vi "Tosca-Editor.vi"(0 "Tosca":refnum<class "Parameters.lvclass">, 2 "Parent VI":refnum<vi>, 5 "FSM In":refnum<class "FSM.Graph.lvclass">, 9 "Cal Folder":path) -> (4 "Tosca out":refnum<class "Parameters.lvclass">, 6 "FSM out":refnum<class "FSM.Graph.lvclass">, 10 "canceled":bool)   [LabVIEW 2020]
uses:
  FSM Graph VIs/LV Source/FSM Editor/FSM Editor.xctl
  FSM Graph VIs/LV Source/Classes/FSM.Graph/FSM.Graph.lvclass
  Controls/Timeout XCtrl/Timeout XCtrl.xctl
  Classes/Timeout/Timeout.lvclass
  Controls/TTL XCtrl/TTL XCtrl.xctl
  Classes/Parameters/Parameters.lvclass
  Controls/Input Event XCtrl/Input Event XCtrl.xctl
  epl-vi-lib/Utility VIs/Controls/KTable/KTable.xctl
  epl-vi-lib/Utility VIs/Controls/KListboxEx/KListboxEx.xctl
  Controls/Termination XCtrl/Termination XCtrl.xctl
  Classes/Termination/Termination.lvclass
  epl-vi-lib/Signal Synthesis VIs/4th Generation/Controls/SignalManager/SignalManager.xctl
  epl-vi-lib/Signal Synthesis VIs/4th Generation/Classes/SignalManager/SignalManager.lvclass
  Classes/Parameters/Parameters.lvclass/Parameters.ctl
  Typedefs/Tosca-Schedule Mode.ctl
  Classes/State/State.lvclass/State.ctl
  FSM Graph VIs/LV Source/Classes/FSM.Node/Badge.ctl
  epl-vi-lib/Signal Synthesis VIs/4th Generation/Classes/SignalManager/SignalManager.lvclass/SignalManager.ctl
  Classes/Timeout/Timeout.lvclass/Timeout.ctl
  Classes/Termination/Termination.lvclass/Termination.ctl
  Classes/Parameters/Read Flowchart.vi
  Classes/Parameters/Write DAQ.vi
  Classes/Parameters/Write Schedule Mode.vi
  Classes/Parameters/Read Input Events.vi
  Classes/Parameters/Read Flags.vi
  Classes/State/Read Name.vi
  Classes/Parameters/Write First state.vi
  Classes/Parameters/Write Target state.vi
  epl-vi-lib/Signal Synthesis VIs/4th Generation/Classes/SignalManager/Read Fs (Hz).vi
  Classes/Parameters/Read Pretrial.vi
  Classes/Parameters/Read DAQ.vi
  Classes/Parameters/Read Schedule Mode.vi
  Classes/State/Read Timeouts.vi
  Classes/Timeout/Read Link to.vi
  Classes/Timeout/Read Type.vi
  epl-vi-lib/Signal Synthesis VIs/4th Generation/Classes/SignalManager/Read Error.vi
  Classes/State/Read script.vi
  Classes/State/Read TTL-only.vi
  Classes/State/Read SigMan.vi
  Classes/State/Read Grating.vi
  Classes/Parameters/Read First state.vi
  Classes/Parameters/Read Target state.vi
  Classes/Timeout/Read TTL.vi
  Classes/State/Read Term.vi
  Classes/Termination/Read TTL.vi
  Classes/Termination/Read Source.vi
  Classes/Termination/Read Type.vi
  Sub VIs/Tosca-Globals.vi
  Classes/State/State.lvclass
  TTL VIs/Control Classes/Base Class/TTLController.lvclass
  FSM Graph VIs/LV Source/Classes/FSM.Node/FSM.Node.lvclass
panel:
  in  "Template":u16(ring) items=["Create from template...", "Basic"]
  in  "FSM.Graph":refnum<class "FSM.Graph.lvclass">(xcontrol)
  in  "Cancel":bool
  in  "Apply":bool
  in  "Tabs":T1(tab)
  in  "icon":u16(ring)
  in  "Mode":u16(ring) caption="Configure as" items=["Sequence", "CS+/CS-", "Adaptive track"]
  in  "DAQ":T2
  in  "Input Event":T6(xcontrol)
  in  "Flags":u16(xcontrol)
  in  "EventList":i32(xcontrol) caption="Input event..."
  in  "State.Script":bool caption="Re-execute script"
  in  "Time/Term":enum32{"Timeout", "Term"}(tab)
  in  "Timeout":refnum<class "Timeout.lvclass">(xcontrol)
  in  "Term":refnum<class "Termination.lvclass">(xcontrol) caption="Lick"
  in  "State.Target":bool caption="Target state"
  in  "State.Start here":bool caption="Start here"
  in  "State.Name":string caption="Name"
  in  "TTL":refnum<class "TTLController.lvclass">[](xcontrol)
  in  "SigMan":refnum<class "SignalManager.lvclass">(xcontrol)
  in  "Sig Tab":enum32{"Error", "Plot"}(tab)
  out "Error":string
  out "Graph":dbl[][](graph)
  in  "Grating":T7
  in  "Test Button":bool
  # "delay between starting locomotion tracking, \nSynapse, etc. and before starting first trial"
  # "Events evaluated in this order.\nDrag to rearrange"
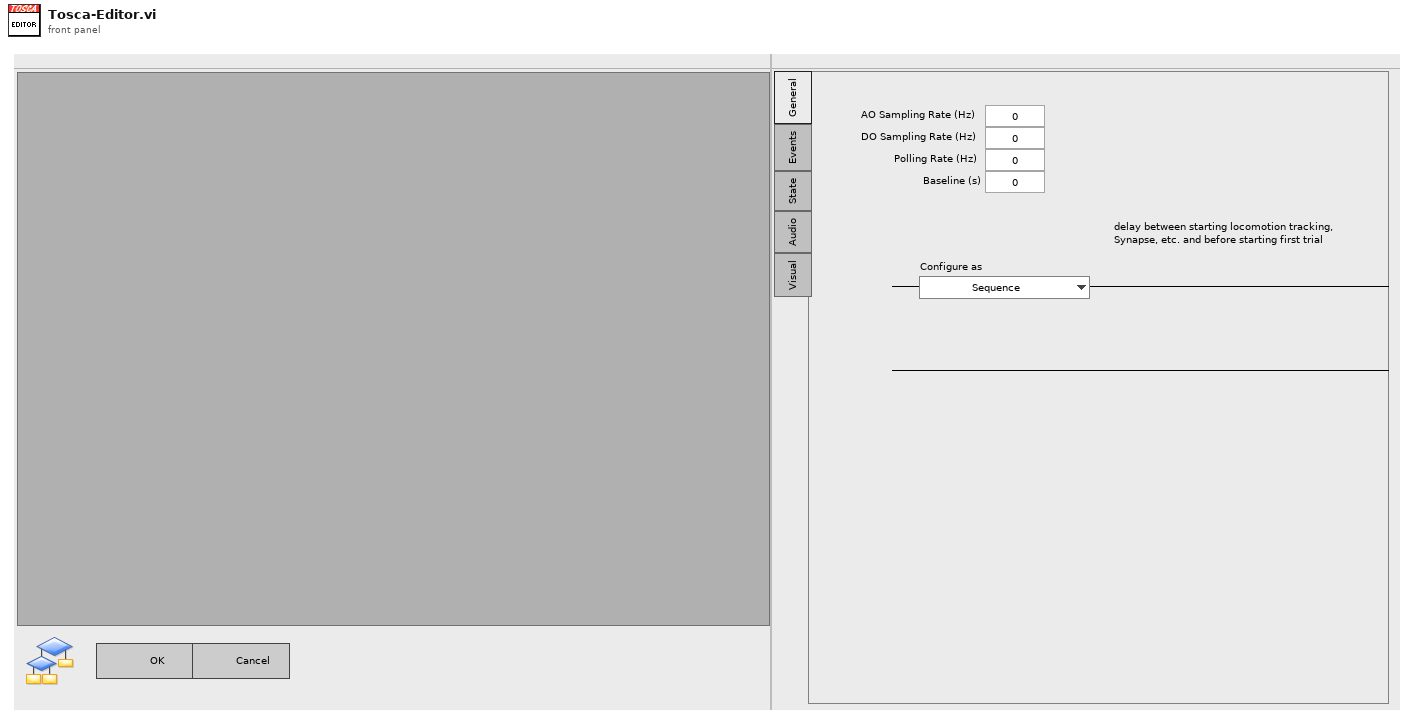
[diagram p1: front panel]
types:
  T1 = enum32{"General", "Events", "State", "Audio", "Visual"}
  T2 = cluster{"AO Sampling Rate (Hz)":dbl, "DO Sampling Rate (Hz)":dbl, "Polling Rate (Hz)":dbl, "Baseline (s)":dbl}
  T3 = typedef "Tosca-Input Criterion.ctl" = cluster{"DigInput":i32, "State":T4, "Time (ms)":i32, "Name":string}
  T4 = typedef "Logic State.ctl" = enum16{"Low", "High", "Rising", "Falling"}
  T5 = typedef "Tosca-Accumulator.ctl" = cluster{"active":bool, "N":i32, "T":dbl, "Imax":dbl, "latency":dbl}
  T6 = cluster{"Name":string, "Criteria":T3[], "Operators":enum16{"AND", "OR"}[], "Accumulator":T5}
  T7 = cluster{"Grating type":enum16{"OFF", "Square", "Sine"}, "Orientation (degrees)":dbl, "Spatial frequency (cpd)":dbl, "Velocity (Hz)":dbl, "Contrast (0-1)":dbl, "Mean intensity (0-1)":dbl, "Duration (ms)":dbl, "Phase (cycles)":dbl}
  T8 = cluster{"selectedState":i32, "selectedTrans":i32, "termSelected":bool, "selectedEvent":i32}
  T9 = typedef "Tosca-Schedule Mode.ctl" = enum16{"Seq", "CS+/CS-", "Adapt"}
  T10 = enum32{"Input Events", "Schedule", "State", "Audio", "Visual"}
  T11 = enum8{"Enabled", "Disabled", "Disabled and Grayed Out"}
  T12 = typedef "FSM.Node.lvclass/Badge.ctl" = enum16{"Audio", "Visual"}
  T13 = typedef "KListboxEx.xctl/Event Action.ctl" = enum16{"None", "Add", "Delete", "Move", "Edit", "Select"}
  T14 = typedef "Tosca-Input Event.ctl" = cluster{"Name":string, "Criteria":T3[], "Operators":enum16{"AND", "OR"}[], "Accumulator":T5}
  T15 = typedef "Tosca-Flag.ctl" = cluster{"Name":string, "Default":i32}
  T16 = typedef "FSM.Annotation.lvclass/Annotation Style.ctl" = enum16{"Plain", "On", "Off", "On-Off"}
  T17 = typedef "Tosca-Visual Display Settings.ctl" = cluster{"Use PTB":bool, "IP Address":string, "Port":i32, "rect":cluster{"left":i16, "top":i16, "width":i16, "height":i16}, "Full screen":bool, "Open at start":bool, "Monitor":i32, "Monitor size (in)":dbl, "Monitor dist (in)":dbl, "Photodiode Square":cluster{"size":i16, "location":enum16{"Bottom Left", "Top Left", "Top Right", "Bottom Right"}}, "Background":dbl}
  T18 = typedef "Parameters.lvclass/DAQ.ctl" = cluster{"AO Fs (Hz)":dbl, "DO Fs (Hz)":dbl, "Poll Rate (Hz)":dbl, "Baseline (s)":dbl}
  T19 = typedef "Tosca-Pretrial Spec.ctl" = cluster{"Path":path, "Args":string[]}
  T20 = typedef "Tosca-Event Type.ctl" = enum16{"Normal", "CS+", "CS-"}
  T21 = typedef "Tosca-Grating.ctl" = cluster{"Type":T22, "Orientation (deg)":dbl, "Spatial frequency (cpd)":dbl, "Velocity (Hz)":dbl, "Contrast":dbl, "Background intensity":dbl, "Duration (ms)":dbl, "Phase (cycles)":dbl}
  T22 = typedef "Tosca-Grating Type.ctl" = enum16{"OFF", "Square", "Sine"}
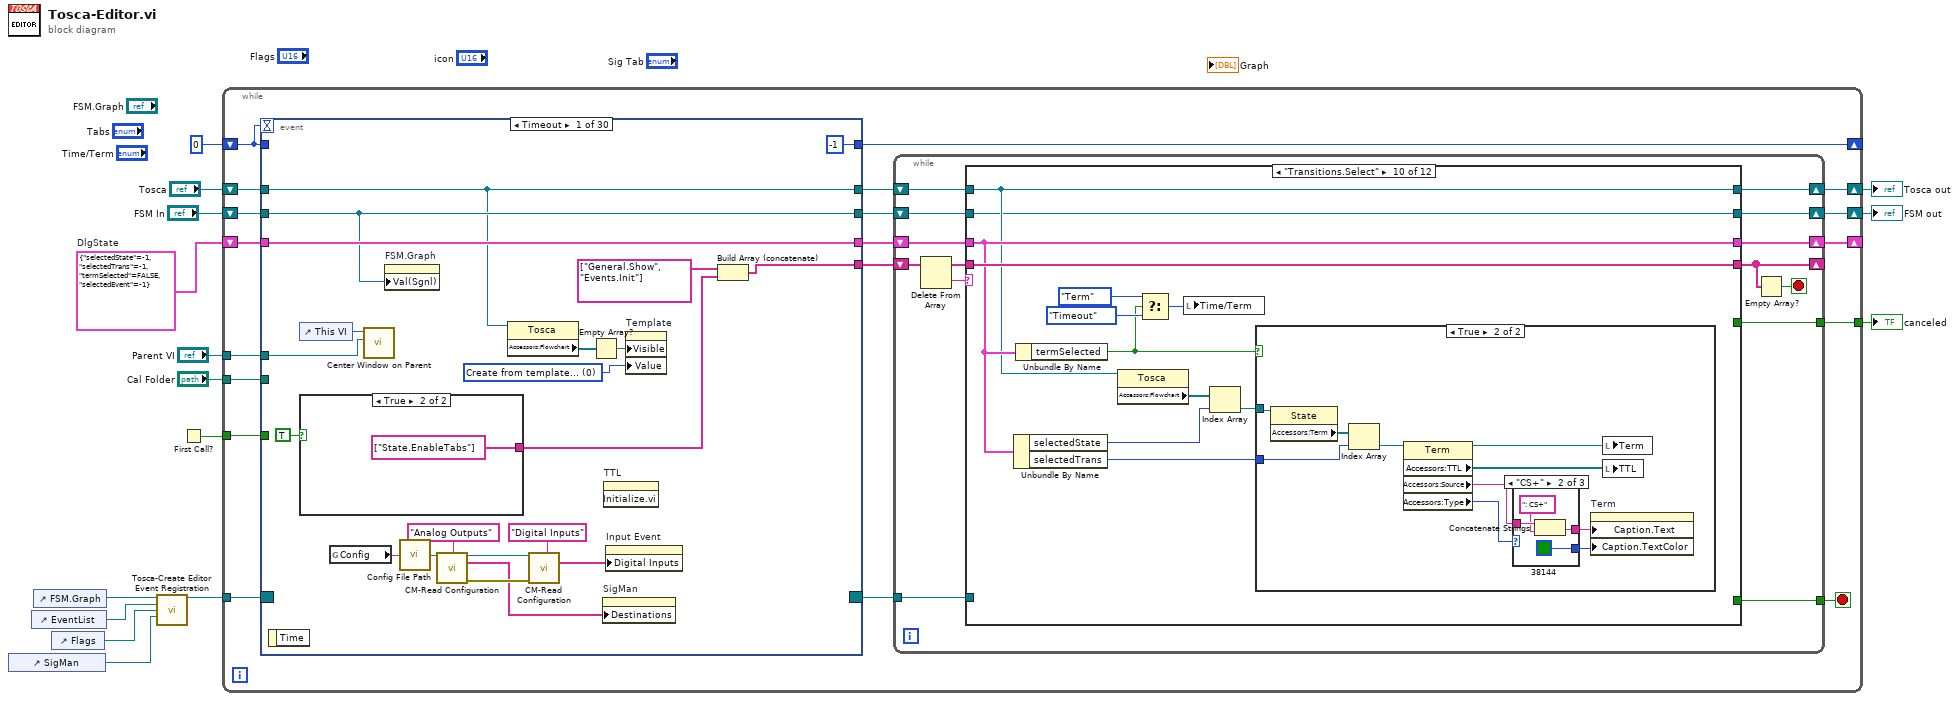
[diagram p0: block diagram]
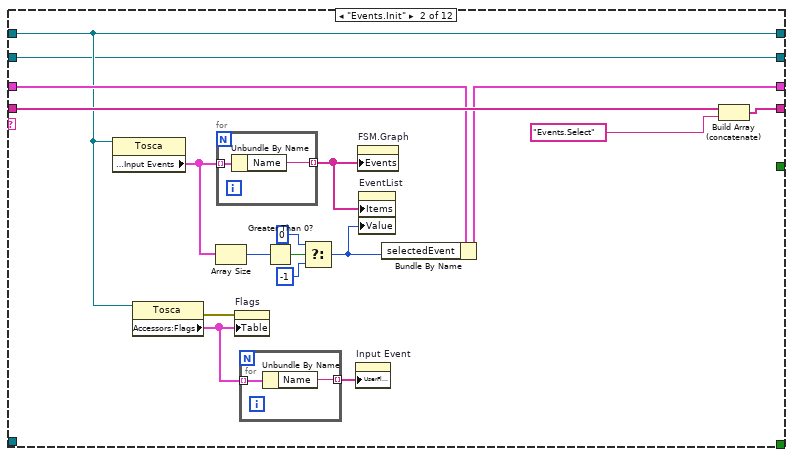
[diagram p3: hidden frame]
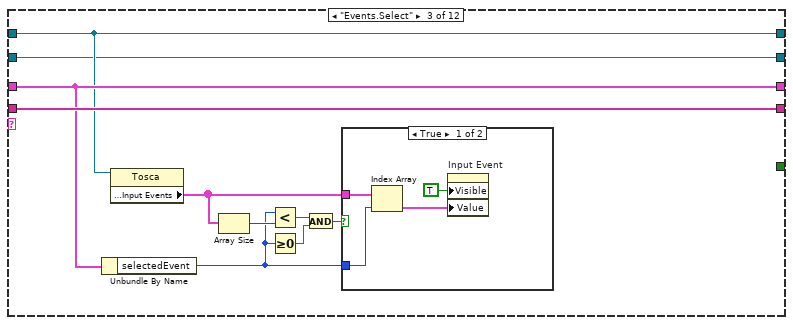
[diagram p4: hidden frame]
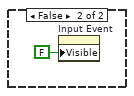
[diagram p5: hidden frame]
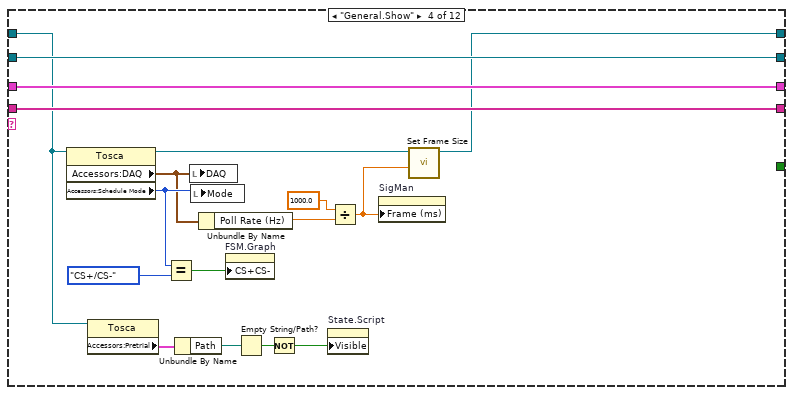
[diagram p6: hidden frame]
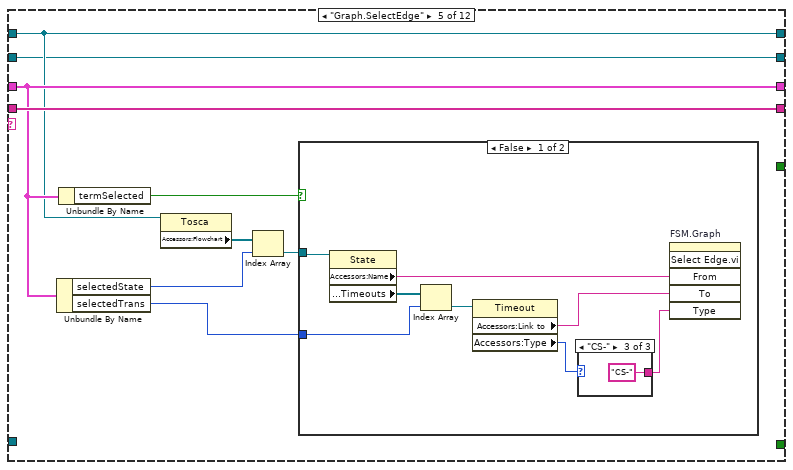
[diagram p7: hidden frame]
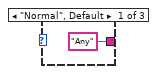
[diagram p8: hidden frame]
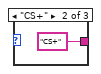
[diagram p9: hidden frame]
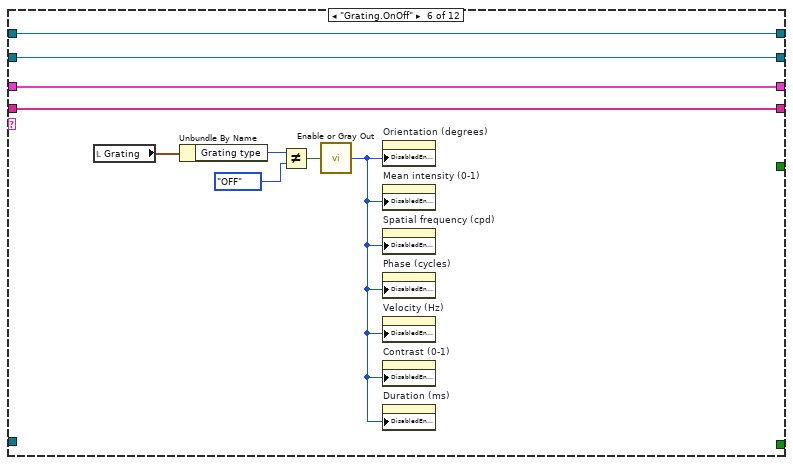
[diagram p11: hidden frame]
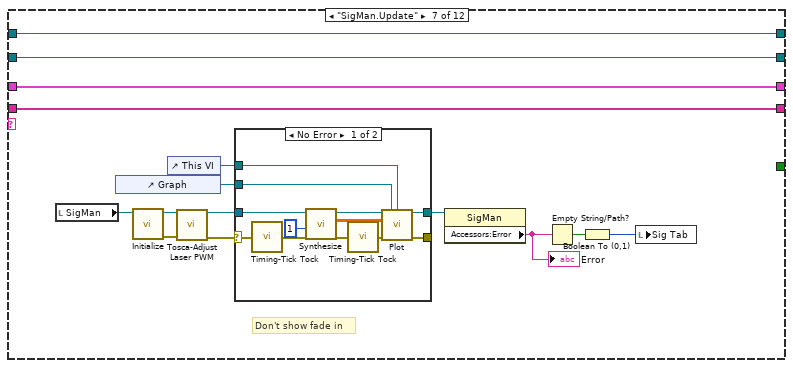
[diagram p12: hidden frame]
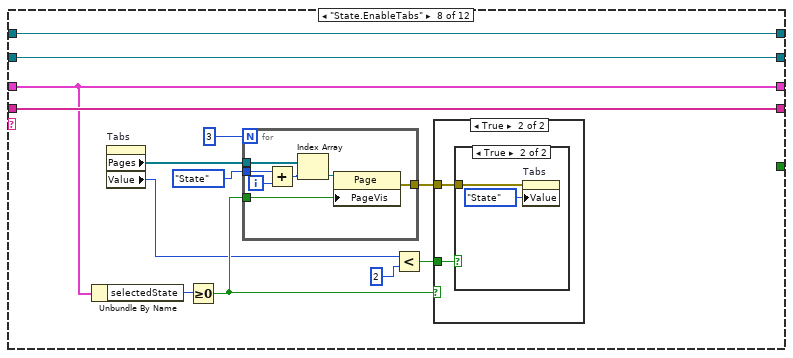
[diagram p14: hidden frame]
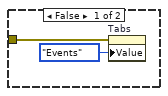
[diagram p15: hidden frame]
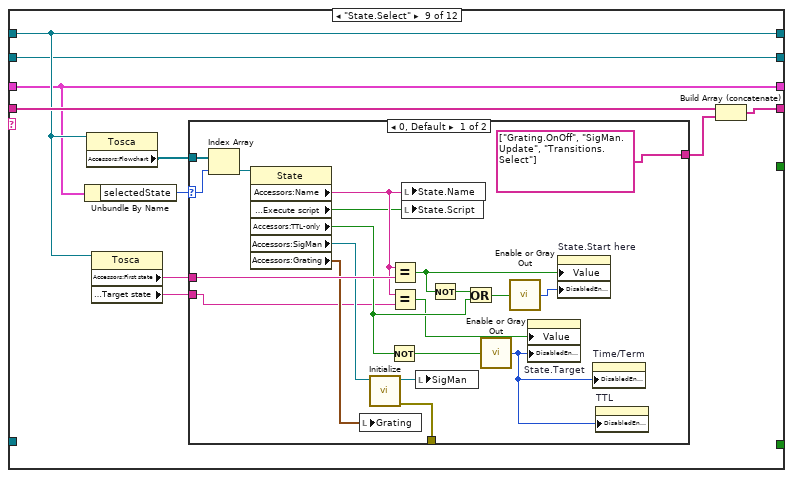
[diagram p17: hidden frame]
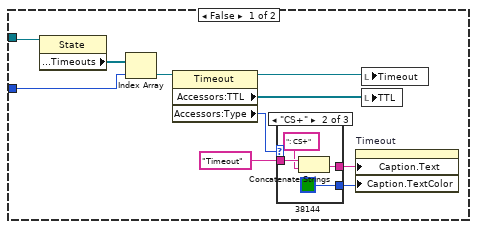
[diagram p19: hidden frame]
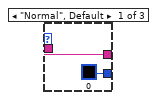
[diagram p20: hidden frame]
diagram:
  w13 = T8 {"selectedState"=-1, "selectedTrans"=-1, "termSelected"=FALSE, "selectedEvent"=-1}  # DlgState
  n1 = control-ref of="SigMan"() -> (w3:refnum<vi>)
  n2 = control-ref of="EventList"() -> (w10:refnum<vi>)
  n3 = control-ref of="FSM.Graph"() -> (w11:refnum<vi>)
  n4 = control-ref of="Flags"() -> (w9:refnum<vi>)
  n5 = call "Tosca-Create Editor Event Registration.vi"("FSM.Editor Ref"=w11, "EventList Ref"=w10, "Flags Ref"=w9, "SigMan Ref"=w3) -> ("Event Registration Refnum"=w14:refnum<event-registration>)  [unwired: 11 in]
  n6 = First Call?() -> (First Call?: T/F=w12:bool)
  n7 = while {
    shift-right: [w33] -> _
    shift-left: 0 -> [w34]
    shift-right: [w29] -> w8
    shift-left: "Tosca" -> [w32]
    tunnel: w14 -> [w22]
    shift-right: [w26] -> _
    shift-left: w13 -> [w27]
    tunnel: w12 -> [w24]
    shift-right: [w19] -> w7
    shift-left: "FSM In" -> [w21]
    tunnel: [w18] -> w6
    tunnel: "Parent VI" -> [w17]
    tunnel: "Cal Folder" -> [w16]
    stop <- w28 stop-if-true
    n8 = event shown="[0] Timeout" {
      selector: w22 -> [_ _ _ _ _ _ _ _ _ _ _ _ _ _ _ _ _ _ _ _ _ _ _ _ _ _ _ _ _ _]
      dyn-events: [_ _ _ _ _ _ _ _ _ _ _ _ _ _ _ _ _ _ _ _ _ _ _ _ _ _ _ _ _ _] -> w23
      timeout: w34 -> [_ _ _ _ _ _ _ _ _ _ _ _ _ _ _ _ _ _ _ _ _ _ _ _ _ _ _ _ _ _]
      tunnel: w34 -> [_ w310 w317 w322 w328 w334 w342 w350 w361 w401 w408 w419 w430 w445 w455 w462 w470 w482 w496 w522 w534 w562 w569 w584 w595 w609 w623 w635 w642 w653]
      tunnel: [-1 w310 w317 w322 w328 w334 w342 w350 w361 w401 w408 w419 w430 w445 w455 w462 w470 w482 w496 w522 w534 w562 w569 w584 w595 w609 w623 w635 w642 w653] -> w33
      tunnel: w32 -> [w295 w311 w316 w321 w326 w331 w336 w348 w356 w400 w404 w415 w428 w439 w451 w459 w468 w480 w491 w514 w531 w561 w567 w583 w588 w607 w614 w633 w637 w648]
      tunnel: [w295 w311 w316 w321 w325 w330 w335 w347 w355 w400 w403 w412 w427 w435 w447 w458 w464 w477 w490 w513 w530 w561 w565 w583 w587 w605 w614 w632 w636 w646] -> w31
      tunnel: [w301 string[] ["cancel"] string[] ["cancel"] string[] ["ok"] _ _ _ _ w352 string[] ["Events.Select"] _ _ _ _ _ _ _ w472 _ string[] ["SigMan.Update"] string[] ["Grating.OnOff"] _ _ string[] ["Graph.SelectEdge", "State.EnableTabs", "State.Select"] string[] ["State.EnableTabs", "State.Select"] string[] ["Transitions.Select"] string[] ["State.Select", "State.EnableTabs"] string[] ["State.Select"] _ w644] -> w30
      tunnel: w27 -> [w304 w308 w314 w319 w327 w333 w341 w349 w354 w399 w407 w418 w429 w444 w454 w460 w469 w481 w495 w521 w533 w560 w568 w582 w594 w608 w622 w634 w641 w652]
      tunnel: [w304 w308 w314 w319 w327 w333 w341 w349 w353 w398 w407 w418 w429 w444 w454 w460 w469 w481 w495 w521 w533 w560 w568 w581 w593 w600 w618 w627 w641 w652] -> w25
      tunnel: w24 -> [_ _ _ _ _ _ _ _ _ _ _ _ _ _ _ _ _ _ _ _ _ _ _ _ _ _ _ _ _ _]
      tunnel: w21 -> [w296 w307 w313 w318 w324 w332 w340 w343 w351 w395 w402 w409 w422 w434 w446 w461 w463 w471 w487 w516 w523 w559 w564 w570 w589 w596 w610 w624 w640 w647]
      tunnel: [w296 w307 w313 w318 w324 w332 w340 w343 w351 w395 w402 w409 w422 w434 w446 w461 w463 w471 w487 w516 w523 w559 w564 w570 w589 w596 w610 w624 w640 w645] -> w20
      tunnel: w17 -> [w298 _ _ _ _ _ _ _ _ _ _ _ _ _ _ _ _ _ _ _ _ _ _ _ _ _ _ _ _ _]
      tunnel: w16 -> [_ _ _ _ _ _ _ _ _ _ _ _ _ _ _ _ _ _ _ _ _ _ w563 _ _ _ _ _ _ _]
      event Timeout {
        w292 = u16 0 items=["Create from template...", "Basic"] ("Template")
        n9 = event-data() -> ()  [unwired: 1 in, 1 out]
        n10 = control-ref of="This VI"() -> (w299:refnum<vi>)
        n11 = case shown="True" TRUE {
          tunnel: [_ string[] ["State.EnableTabs"]] -> w302
          frame False {
          }
          frame True {
          }
        }
        n12 = global read "Tosca-Globals.vi" "Config"() -> (w303:string)
        n13 = call "Center Window on Parent.vi"("Parent VI"=w298, "VI in"=w299) -> ()  [unwired: 8 in, 2 out]
        n14 = property on="FSM.Graph" class="FSMGraph (strict)"("Val(Sgnl)"=w296) -> ()  [unwired: 2 in, 2 out]
        n15 = call "Config File Path.vi"("AppName"=w303) -> ("Default config file name"=w288:path)
        n16 = call "CM-Read Configuration.vi"("Connection File Path"=w288, "Section"="Analog Outputs") -> ("Connection File Path thru"=w287:path, "Names"=w285:string[], "error out"=w286:errorcluster)  [unwired: 9 in, 2 out]
        n17 = property on="Property Node" class="Tosca"(reference=w295) -> ("Accessors:Flowchart"=w294:refnum<class "State.lvclass">[])  [unwired: 1 in, 2 out]
        n18 = call "CM-Read Configuration.vi"("Connection File Path"=w287, "Section"="Digital Inputs", "error in (no error)"=w286) -> ("Names"=w290:string[])  [unwired: 8 in, 4 out]
        n19 = Empty Array?(array=w294) -> (empty?=w293:bool)
        n20 = property on="SigMan" class="SignalManager (strict)"("Destinations"=w285) -> ()  [unwired: 2 in, 2 out]
        n21 = invoke on="TTL" class="TTL XCtrl (strict)" method="Initialize.vi"() -> ()  [unwired: 3 in, 3 out]
        n22 = property on="Input Event" class="Input Event XCtrl (strict)"("Digital Inputs"=w290) -> ()  [unwired: 2 in, 2 out]
        n23 = property on="Template" class="Ring (strict)"("Visible"=w293, "Value"=w292) -> ()  [unwired: 2 in, 2 out]
        n24 = Build Array (concatenate)(string[] ["General.Show", "Events.Init"], w302) -> (w301:string[])
      }
      event Panel Close? {
        n25 = event-data() -> ()  [unwired: 1 in, 1 out]
        n26 = event-data("Discard?"=TRUE) -> ()  [unwired: 1 in, 1 out]
      }
      event "Cancel": Value Change {
        n27 = event-data() -> ()  [unwired: 1 in, 1 out]
      }
      event "Apply": Value Change {
        n28 = event-data() -> ()  [unwired: 1 in, 1 out]
      }
      event "DAQ": Value Change {
        n29 = event-data() -> ()  [unwired: 1 in, 1 out]
        n30 = property class="Tosca"(reference=w326, "Accessors:DAQ"="DAQ") -> (reference out=w325:refnum<class "Parameters.lvclass">)  [unwired: 1 in, 1 out]
      }
      event "DAQ.AO Sampling Rate (Hz)": Value Change {
        n31 = event-data() -> ("NewVal"=w329:dbl)  [unwired: 1 in]
        n32 = property on="SigMan" class="SignalManager (strict)"("Fs (Hz)"=w329) -> ()  [unwired: 2 in, 2 out]
        n33 = call "Set AO Sampling Rate.vi"("Fs (Hz)"=w329, "Tosca in"=w331) -> ("Tosca out"=w330:refnum<class "Parameters.lvclass">)  [unwired: 8 in, 1 out]
      }
      event "DAQ.Polling Rate (Hz)": Value Change {
        n34 = event-data() -> ("NewVal"=w339:dbl)  [unwired: 1 in]
        n35 = Divide(x=1000.0, y=w339) -> (x/y=w338:dbl)
        n36 = property on="SigMan" class="SignalManager (strict)"("Frame (ms)"=w338) -> ()  [unwired: 2 in, 2 out]
        n37 = call "Set Frame Size.vi"("Frame (ms)"=w338, "Tosca in"=w336) -> ("Tosca out"=w335:refnum<class "Parameters.lvclass">)  [unwired: 8 in, 1 out]
      }
      event "Mode": Value Change {
        n38 = event-data() -> ()  [unwired: 1 in, 1 out]
        n39 = Equal?(x="Mode", y=Tosca-Schedule_Mode."CS+/CS-" ("Schedule Mode")) -> (x = y?=w345:bool)
        n40 = property class="Tosca"(reference=w348, "Accessors:Schedule Mode"="Mode") -> (reference out=w347:refnum<class "Parameters.lvclass">)  [unwired: 1 in, 1 out]
        n41 = property on="FSM.Graph" class="FSMGraph (strict)"("CS+CS-"=w345) -> ()  [unwired: 2 in, 2 out]
      }
      event User Event {
        n42 = event-data() -> ("Action"=w360:T13, "Name"=w359:string, "Start row"=w358:i32, "End row"=w357:i32)  [unwired: 1 in]
        n43 = case shown="\"Add\"" w360 {
          tunnel: w359 -> [_ w370 w374 _ _]
          tunnel: w358 -> [_ w368 w377 w381 w393]
          tunnel: w357 -> [_ _ _ _ w392]
          tunnel: w356 -> [w363 w371 w379 w389 w391]
          tunnel: [w363 w364 w378 w388 w390] -> w355
          tunnel: w354 -> [w362 w369 w380 w385 w394]
          tunnel: [w362 w369 w380 w384 w394] -> w353
          tunnel: [_ _ string[] ["State.Select"] string[] ["State.Select"] _] -> w352
          frame "None", Default {
          }
          frame "Add" {
            n44 = call "Add Event.vi"("Insert At"=w368, "Name"=w370, "Tosca in"=w371) -> ("Tosca out"=w365:refnum<class "Parameters.lvclass">)  [unwired: 7 in, 1 out]
            n45 = property class="Tosca"(reference=w365) -> (reference out=w364:refnum<class "Parameters.lvclass">, "Accessors:Input Events"=w367:T14[])  [unwired: 1 in, 1 out]
            n46 = for {
              tunnel: w367 -> [w373] mode=indexing
              tunnel: [w372] -> w366 mode=indexing
              n47 = Unbundle By Name(w373) -> ("Name"=w372:string)
            }
            n48 = property on="FSM.Graph" class="FSMGraph (strict)"("Events"=w366) -> ()  [unwired: 2 in, 2 out]
          }
          frame "Edit" {
            n49 = call "Rename Event.vi"("eventIndex"=w377, "Name"=w374, "Tosca in"=w379) -> ("Old Name"=w375:string, "Tosca out"=w378:refnum<class "Parameters.lvclass">)  [unwired: 6 in, 1 out]
            n50 = invoke on="FSM.Graph" class="FSM Editor (strict)" method="Rename Edges.vi"("Old Name"=w375, "New Name"=w374) -> ()  [unwired: 3 in, 5 out]
          }
          frame "Delete" {
            n51 = call "Delete Event.vi"("DeleteAt"=w381, "Tosca in"=w389) -> ("Name"=w387:string, "Tosca out"=w388:refnum<class "Parameters.lvclass">)  [unwired: 7 in, 1 out]
            n52 = Decrement(x=w381) -> ()  [unwired: 1 out]
            n53 = invoke on="FSM.Graph" class="FSM Editor (strict)" method="Delete Edges.vi"("Name"=w387) -> ()  [unwired: 3 in, 4 out]
            n54 = Bundle By Name(cluster=w385, "selectedTrans"=0, "termSelected"=FALSE) -> (w384:T8)
          }
          frame "Move" {
            n55 = call "Move Event.vi"("endIndex"=w392, "startIndex"=w393, "Tosca in"=w391) -> ("Tosca out"=w390:refnum<class "Parameters.lvclass">)  [unwired: 7 in, 1 out]
          }
        }
      }
      event "EventList": Value Change {
        n56 = event-data() -> ()  [unwired: 1 in, 1 out]
        n57 = Bundle By Name(cluster=w399, "selectedEvent"="EventList") -> (w398:T8)
      }
      event "Input Event": Value Change {
        n58 = event-data() -> ()  [unwired: 1 in, 1 out]
        n59 = Unbundle By Name(w407) -> ("selectedEvent"=w405:i32)
        n60 = call "Modify Event.vi"("EventIndex"=w405, "Event"="Input Event", "Tosca in"=w404) -> ("Tosca out"=w403:refnum<class "Parameters.lvclass">)  [unwired: 7 in, 1 out]
      }
      event User Event {
        (unwired) string[] ["Events.Select"]
        n61 = event-data() -> ()  [unwired: 1 in, 1 out]
        n62 = property class="Tosca" props=["Accessors:Flags", "Accessors:Input Events"](reference=w415) -> (reference out=w413:refnum<class "Parameters.lvclass">, "Accessors:Flags"=w416:T15[])  [unwired: 1 in, 2 out]
        n63 = invoke on="Flags" class="KTable (strict)" method="Read Table.vi"("Type of Anything"=w416) -> ("Read Table.vi"=w417:variant)  [unwired: 3 in, 3 out]
        n64 = Variant To Data(type=w416, Variant=w417) -> (data=w411:T15[])  [unwired: 1 in, 1 out]
        n65 = for {
          tunnel: w411 -> [w421] mode=indexing
          tunnel: [w420] -> w414 mode=indexing
          n66 = Unbundle By Name(w421) -> ("Name"=w420:string)
        }
        n67 = call "Update Flags.vi"("Flags"=w411, "Tosca in"=w413) -> ("error out"=w410:errorcluster, "Tosca out"=w412:refnum<class "Parameters.lvclass">)  [unwired: 8 in]
        n68 = property on="Input Event" class="Input Event XCtrl (strict)"(error in=w410, "UserFlags"=w414) -> ()  [unwired: 1 in, 2 out]
      }
      event "State.Name": Value Change {
        n69 = event-data() -> ("NewVal"=w425:string, "OldVal"=w423:string)  [unwired: 1 in]
        n70 = Unbundle By Name(w429) -> ("selectedState"=w424:i32)
        n71 = call "Rename State.vi"("Tosca in"=w428, "stateIndex"=w424, "New name"=w425) -> ("Tosca out"=w427:refnum<class "Parameters.lvclass">, "accepted"=w426:bool)  [unwired: 11 in]
        n72 = case shown="True" w426 {
          tunnel: w425 -> [_ w433]
          tunnel: w424 -> [_ w432]
          tunnel: w423 -> [w431 _]
          frame False {
            n73 = local write "State.Name"(w431) -> ()
          }
          frame True {
            n74 = invoke on="FSM.Graph" class="FSM Editor (strict)" method="Rename Node.vi"("Index"=w432, "New name"=w433) -> ()  [unwired: 3 in, 5 out]
          }
        }
      }
      event "State.Start here": Value Change {
        n75 = event-data() -> ("CtlRef"=w441:refnum<vi>)  [unwired: 1 in]
        n76 = Unbundle By Name(w444) -> ("selectedState"=w442:i32)
        n77 = property class="Tosca"(reference=w439) -> (reference out=w437:refnum<class "Parameters.lvclass">, "Accessors:Flowchart"=w438:refnum<class "State.lvclass">[])  [unwired: 1 in, 1 out]
        n78 = property class="Bool (strict)"(reference=w441, "DisabledEnum"=T11."Disabled and Grayed Out" ("Disabled")) -> ()  [unwired: 1 in, 2 out]
        n79 = Index Array(array=w438, index=w442) -> (element=w443:refnum<class "State.lvclass">)
        n80 = property class="State"(reference=w443) -> ("Accessors:Name"=w436:string)  [unwired: 1 in, 2 out]
        n81 = invoke on="FSM.Graph" class="FSM Editor (strict)" method="Set Start Node.vi"("Index"=w442) -> ()  [unwired: 3 in, 4 out]
        n82 = property class="Tosca"(reference=w437, "Accessors:First state"=w436) -> (reference out=w435:refnum<class "Parameters.lvclass">)  [unwired: 1 in, 1 out]
      }
      event "State.Target": Value Change {
        n83 = event-data() -> ()  [unwired: 1 in, 1 out]
        n84 = Unbundle By Name(w454) -> ("selectedState"=w452:i32)
        n85 = property class="Tosca"(reference=w451) -> (reference out=w449:refnum<class "Parameters.lvclass">, "Accessors:Flowchart"=w450:refnum<class "State.lvclass">[])  [unwired: 1 in, 1 out]
        n86 = Index Array(array=w450, index=w452) -> (element=w453:refnum<class "State.lvclass">)
        n87 = invoke on="FSM.Graph" class="FSM Editor (strict)" method="Set Target Node.vi"("Index"=w452) -> ()  [unwired: 3 in, 4 out]
        n88 = property class="State"(reference=w453) -> ("Accessors:Name"=w448:string)  [unwired: 1 in, 2 out]
        n89 = property class="Tosca"(reference=w449, "Accessors:Target state"=w448) -> (reference out=w447:refnum<class "Parameters.lvclass">)  [unwired: 1 in, 1 out]
      }
      event "State.Script": Value Change {
        n90 = event-data() -> ()  [unwired: 1 in, 1 out]
        n91 = Unbundle By Name(w460) -> ("selectedState"=w457:i32)
        n92 = call "Set Execute Script.vi"("Tosca in"=w459, "stateIndex"=w457, "Execute script"="State.Script") -> ("Tosca out"=w458:refnum<class "Parameters.lvclass">)  [unwired: 11 in, 1 out]
      }
      event "Timeout": Value Change {
        n93 = event-data() -> ()  [unwired: 1 in, 1 out]
        n94 = Unbundle By Name(w469) -> ("selectedState"=w466:i32, "selectedTrans"=w465:i32)
        n95 = call "Set Timeout.vi"("Tosca in"=w468, "Timeout"="Timeout", "stateIndex"=w466, "timeOut Index"=w465) -> ("Tosca out"=w464:refnum<class "Parameters.lvclass">)  [unwired: 10 in, 1 out]
      }
      event "Term": Value Change {
        n96 = event-data() -> ()  [unwired: 1 in, 1 out]
        n97 = Unbundle By Name(w481) -> ("selectedState"=w479:i32, "selectedTrans"=w478:i32)
        n98 = call "Set Termination.vi"("Tosca in"=w480, "Termination"="Term", "stateIndex"=w479, "termIndex"=w478) -> ("Tosca out"=w477:refnum<class "Parameters.lvclass">, "change action state"=w473:i32, "TTL-only"=w474:bool, "error out"=w475:errorcluster)  [unwired: 8 in]
        n99 = case shown="0, Default" w473 {
          selector: w473 -> [w486 _]
          tunnel: w474 -> [w485 _]
          frame 0, Default {
            n100 = invoke on="FSM.Graph" class="FSM Editor (strict)" method="Set Action-only.vi"("Index"=w486, "action-only"=w485) -> ()  [unwired: 3 in, 5 out]
          }
          frame -1 {
          }
        }
        n101 = case shown="Error" w475 {
          selector: w475 -> [_ w484]
          tunnel: [_ string[] ["State.Select"]] -> w472
          frame No Error {
          }
          frame Error {
            n102 = call "Error Handler.vi"("error in (no error)"=w484) -> ()  [unwired: 12 in, 3 out]
          }
        }
      }
      event "TTL": Value Change {
        n103 = event-data() -> ()  [unwired: 1 in, 1 out]
        n104 = invoke on="FSM.Graph" class="FSM Editor (strict)" method="Clear Annotations.vi"() -> (error out=w488:errorcluster)  [unwired: 3 in, 2 out]
        n105 = Unbundle By Name(w495) -> ("selectedState"=w492:i32, "selectedTrans"=w493:i32, "termSelected"=w494:bool)
        n106 = case shown="False" w494 {
          tunnel: w493 -> [w501 w506]
          tunnel: w492 -> [w502 w507]
          tunnel: "TTL" -> [w503 w508]
          tunnel: [w504 w509] -> w490
          tunnel: w491 -> [w505 w510]
          frame False {
            n107 = call "Set Timeout TTL.vi"("Tosca in"=w505, "TTL"=w503, "stateIndex"=w502, "timeOut Index"=w501) -> ("Tosca out"=w504:refnum<class "Parameters.lvclass">)  [unwired: 10 in, 1 out]
          }
          frame True {
            n108 = call "Set Termination TTL.vi"("Tosca in"=w510, "TTL"=w508, "stateIndex"=w507, "termIndex"=w506) -> ("Tosca out"=w509:refnum<class "Parameters.lvclass">)  [unwired: 10 in, 1 out]
          }
        }
        n109 = for {
          tunnel: "TTL" -> [w500] mode=indexing
          tunnel: w488 -> [w497]
          n110 = call "Get Annotation Style.vi"("TTLControl in"=w500) -> ("Name"=w499:string, "Style"=w498:T16)  [unwired: 10 in, 3 out]
          n111 = invoke on="FSM.Graph" class="FSM Editor (strict)" method="Add Annotation.vi"(error in=w497, "Name"=w499, "Style"=w498) -> ()  [unwired: 2 in, 5 out]
        }
      }
      event "SigMan": Value Change {
        n112 = event-data() -> ()  [unwired: 1 in, 1 out]
        n113 = Unbundle By Name(w521) -> ("selectedState"=w518:i32)
        n114 = call "Set Signal Manager.vi"("Tosca in"=w514, "stateIndex"=w518, "SigMan"="SigMan") -> ("Tosca out"=w511:refnum<class "Parameters.lvclass">)  [unwired: 11 in, 1 out]
        n115 = property class="SigMan"(reference="SigMan") -> ("Accessors:Fs (Hz)"=w515:dbl)  [unwired: 1 in, 2 out]
        n116 = call "In Use.vi"("SignalManager in"="SigMan") -> ("In use"=w517:bool)  [unwired: 12 in, 2 out]
        n117 = call "Set AO Sampling Rate.vi"("Fs (Hz)"=w515, "Tosca in"=w511) -> ("Tosca out"=w513:refnum<class "Parameters.lvclass">)  [unwired: 8 in, 1 out]
        n118 = invoke on="FSM.Graph" class="FSM Editor (strict)" method="Set Badge.vi"("stateIndex"=w518, "Badge"=Badge."Audio", "Visible"=w517) -> ()  [unwired: 3 in, 6 out]
        n119 = property on="AO Sampling Rate (Hz)" class="DigNum (strict)"("Value"=w515) -> ()  [unwired: 2 in, 2 out]
      }
      event "Grating": Value Change {
        n120 = event-data() -> ()  [unwired: 1 in, 1 out]
        n121 = Unbundle By Name(w533) -> ("selectedState"=w529:i32)
        n122 = Unbundle By Name("Grating") -> ("Grating type"=w526:enum16{"OFF", "Square", "Sine"})
        n123 = call "Set Grating.vi"("Tosca in"=w531, "stateIndex"=w529, "Grating"="Grating") -> ("Tosca out"=w530:refnum<class "Parameters.lvclass">)  [unwired: 11 in, 1 out]
        n124 = Not Equal?(x=w526, y=enum16{"OFF", "Square", "Sine"}."OFF") -> (x != y?=w524:bool)
        n125 = invoke on="FSM.Graph" class="FSM Editor (strict)" method="Set Badge.vi"("stateIndex"=w529, "Badge"=Badge."Visual", "Visible"=w524) -> ()  [unwired: 3 in, 6 out]
      }
      event "Test Button": Value Change {
        n126 = event-data() -> ()  [unwired: 1 in, 1 out]
        n127 = local read "Grating"() -> (w550:T7)
        n128 = Unbundle By Name(w550) -> ("Grating type"=w557:enum16{"OFF", "Square", "Sine"}, "Orientation (degrees)"=w556:dbl, "Spatial frequency (cpd)"=w555:dbl, "Velocity (Hz)"=w554:dbl, "Contrast (0-1)"=w553:dbl, "Mean intensity (0-1)"=w552:dbl, "Duration (ms)"=w551:dbl, "Phase (cycles)"=w549:dbl)
        n129 = call "Tosca-Restore Visual Display Settings.vi"() -> ("Visual Display Settings"=w548:T17)  [unwired: 14 in, 1 out]
        n130 = Unbundle By Name(w548) -> ("IP Address"=w541:string, "Port"=w540:i32)
        n131 = TCP Open Connection(address=w541, remote port or service name=w540) -> (connection ID=w539:refnum<k5>, error out=w538:errorcluster)  [unwired: 3 in]
        n132 = Format Into String(format string="Buffer:%s:%.4f,%.4f,%.4f,%.4f,%.4f,%.4f,%.4f", w557, w556, w555, w554, w553, w552, w551, w549) -> (resulting string=w537:string)  [unwired: 2 in, 1 out]
        n133 = call "TCP-KO-Send Command.vi"("connection ID"=w539, "Command"=w537, "error in (no error)"=w538) -> ("connection ID out"=w536:refnum<k5>, "error out"=w535:errorcluster)  [unwired: 11 in]
        n134 = call "TCP-KO-Send Command.vi"("connection ID"=w536, "Command"="Draw", "error in (no error)"=w535) -> ("connection ID out"=w547:refnum<k5>, "error out"=w543:errorcluster)  [unwired: 11 in]
        n135 = call "TCP-KO-Send Command.vi"("connection ID"=w547, "Command"="Close", "error in (no error)"=w543) -> ("connection ID out"=w545:refnum<k5>, "error out"=w542:errorcluster)  [unwired: 11 in]
        n136 = TCP Close Connection(connection ID=w545, error in (no error)=w542) -> ()  [unwired: 1 in, 2 out]
      }
      event User Event {
        n137 = event-data() -> ("Name"=w566:string)  [unwired: 1 in]
        n138 = call "Add State.vi"("Name"=w566, "Cal Folder"=w563, "Tosca in"=w567) -> ("Tosca out"=w565:refnum<class "Parameters.lvclass">)  [unwired: 7 in, 1 out]
      }
      event User Event {
        n139 = event-data() -> ("Indices"=w577:i32[])  [unwired: 1 in]
        n140 = Array Size(array=w577) -> (size(s)=w578:i32)
        n141 = Index Array(array=w577) -> (element=w576:i32)  [unwired: 1 in]
        n142 = Equal?(x=w578, y=1) -> (x = y?=w579:bool)
        n143 = Select(t=w576, s=w579, f=-1) -> (s? t:f=w574:i32)
        n144 = Bundle By Name(cluster=w582, "selectedState"=w574, "selectedTrans"=0, "termSelected"=FALSE) -> (w581:T8)
      }
      event User Event {
        n145 = event-data() -> ("Indices"=w586:i32[])  [unwired: 1 in]
        n146 = call "Delete States.vi"("Tosca in"=w588, "stateIndex"=w586) -> ("Tosca out"=w587:refnum<class "Parameters.lvclass">)  [unwired: 13 in]
        n147 = Bundle By Name(cluster=w594, "selectedState"=-1, "selectedTrans"=0, "termSelected"=FALSE) -> (w593:T8)
      }
      event User Event {
        n148 = event-data() -> ("Source"=w604:string, "Target"=w603:string, "Event"=w602:string, "Type"=w601:string)  [unwired: 1 in]
        n149 = call "Add Transition.vi"("Tosca in"=w607, "Source"=w604, "Target"=w603, "Event"=w602, "Type"=w601) -> ("Tosca out"=w606:refnum<class "Parameters.lvclass">)  [unwired: 9 in, 1 out]
        n150 = call "Find Transition.vi"("Tosca in"=w606, "Source"=w604, "Target"=w603, "Event"=w602, "Type"=w601) -> ("Tosca out"=w605:refnum<class "Parameters.lvclass">, "transIndex"=w599:i32, "termination"=w598:bool)  [unwired: 6 in, 2 out]
        n151 = Bundle By Name(cluster=w608, "selectedTrans"=w599, "termSelected"=w598) -> (w600:T8)
      }
      event User Event {
        n152 = event-data() -> ("Source"=w612:string, "Target"=w621:string, "Event"=w620:string, "Type"=w619:string)  [unwired: 1 in]
        n153 = call "Find Transition.vi"("Tosca in"=w614, "Source"=w612, "Target"=w621, "Event"=w620, "Type"=w619) -> ("stateIndex"=w613:i32, "transIndex"=w617:i32, "termination"=w616:bool, "error out"=w611:errorcluster)  [unwired: 6 in, 1 out]
        n154 = call "Error Handler.vi"("error in (no error)"=w611) -> ()  [unwired: 12 in, 3 out]
        n155 = Bundle By Name(cluster=w622, "selectedState"=w613, "selectedTrans"=w617, "termSelected"=w616) -> (w618:T8)
        n156 = invoke on="FSM.Graph" class="FSM Editor (strict)" method="Select Node.vi"("NodeIndex"=w613) -> ()  [unwired: 3 in, 4 out]
      }
      event User Event {
        n157 = event-data() -> ("Source"=w631:string, "Target"=w630:string, "Event"=w629:string, "Type"=w628:string)  [unwired: 1 in]
        n158 = call "Delete Transition.vi"("Tosca in"=w633, "Source"=w631, "Target"=w630, "Event"=w629, "Type"=w628) -> ("Tosca out"=w632:refnum<class "Parameters.lvclass">, "stateIndex"=w625:i32)  [unwired: 8 in, 1 out]
        n159 = Bundle By Name(cluster=w634, "selectedState"=w625) -> (w627:T8)
        n160 = invoke on="FSM.Graph" class="FSM Editor (strict)" method="Select Node.vi"("NodeIndex"=w625) -> ()  [unwired: 3 in, 4 out]
      }
      event User Event {
        n161 = event-data() -> ("Old name"=w639:string, "New name"=w638:string)  [unwired: 1 in]
        n162 = call "Rename Signal in Schedule.vi"("Tosca in"=w637, "Old Name"=w639, "New Name"=w638) -> ("Tosca out"=w636:refnum<class "Parameters.lvclass">)  [unwired: 11 in, 1 out]
      }
      event "Template": Value Change {
        n163 = event-data() -> ()  [unwired: 1 in, 1 out]
        n164 = property on="Template" class="Ring (strict)"() -> ("RingText.Text"=w643:string)  [unwired: 2 in, 2 out]
        n165 = call "Tosca-Create Flowchart From Template.vi"("Name"=w643) -> ("Parameters out"=w650:refnum<class "Parameters.lvclass">, "FSM out"=w649:refnum<class "FSM.Graph.lvclass">, "error out"=w651:errorcluster)  [unwired: 12 in]
        n166 = case shown="No Error" w651 {
          selector: w651 -> [_ w658]
          tunnel: w650 -> [w657 _]
          tunnel: w649 -> [w654 _]
          tunnel: w648 -> [_ w660]
          tunnel: w647 -> [_ w659]
          tunnel: [w657 w660] -> w646
          tunnel: [w654 w659] -> w645
          tunnel: [string[] ["General.Show", "Events.Init"] _] -> w644
          frame No Error {
            n167 = property on="Template" class="Ring (strict)"("Visible"=FALSE) -> ()  [unwired: 2 in, 2 out]
            n168 = property on="FSM.Graph" class="FSMGraph (strict)"("Val(Sgnl)"=w654) -> ()  [unwired: 2 in, 2 out]
          }
          frame Error {
            n169 = call "Error Handler.vi"("error in (no error)"=w658) -> ()  [unwired: 12 in, 3 out]
          }
        }
      }
    }
    n170 = while {
      shift-right: [w45] -> _
      shift-left: w30 -> [w48]
      tunnel: [w41] -> w28
      shift-right: [w42] -> w29
      shift-left: w31 -> [w43]
      shift-right: [w40] -> w26
      shift-left: w25 -> [w39]
      tunnel: w23 -> [w38]
      shift-right: [w36] -> w19
      shift-left: w20 -> [w37]
      tunnel: [w35] -> w18
      stop <- w44 stop-if-true
      n171 = Delete From Array(array=w48) -> (deleted portion=w46:string, array with subset deleted=w47:string[])  [unwired: 2 in]
      n172 = case shown="\"Transitions.Select\"" w46 {
        tunnel: w47 -> [w52 w69 w83 w105 w114 w134 w149 w175 w198 w230 w277 w284]
        tunnel: [w52 w60 w83 w105 w114 w134 w149 w175 w192 w230 w277 w284] -> w45
        tunnel: w43 -> [w51 w58 w81 w99 w112 w132 w148 w173 w195 w225 _ w283]
        tunnel: [w51 w58 w81 w89 w112 w132 w148 w173 w195 w225 w272 w283] -> w42
        tunnel: [_ _ _ _ _ _ _ _ _ _ TRUE TRUE] -> w41
        tunnel: [w50 w67 w82 w104 w113 w133 w147 w174 w193 w229 w275 w281] -> w40
        tunnel: w39 -> [w50 w68 w82 w104 w113 w133 w147 w174 w193 w229 w275 w281]
        tunnel: w38 -> [_ _ _ _ _ _ _ _ _ _ w274 w280]
        tunnel: w37 -> [w49 w53 w74 w103 w106 w126 w141 w163 w190 w219 _ _]
        tunnel: [w49 w53 w74 w103 w106 w126 w141 w163 w190 w219 w271 w278] -> w36
        tunnel: [_ _ _ _ _ _ _ _ _ _ TRUE _] -> w35
        frame "", Default {
        }
        frame "Events.Init" {
          n173 = property class="Tosca"(reference=w58) -> ("Accessors:Input Events"=w66:T14[])  [unwired: 1 in, 2 out]
          n174 = property class="Tosca"(reference=w58) -> (error out=w57:errorcluster, "Accessors:Flags"=w55:T15[])  [unwired: 1 in, 1 out]
          n175 = Array Size(array=w66) -> (size(s)=w63:i32)
          n176 = for {
            tunnel: w66 -> [w73] mode=indexing
            tunnel: [w72] -> w56 mode=indexing
            n177 = Unbundle By Name(w73) -> ("Name"=w72:string)
          }
          n178 = property on="Flags" class="KTable (strict)"(error in=w57, "Table"=w55) -> ()  [unwired: 1 in, 2 out]
          n179 = for {
            tunnel: w55 -> [w71] mode=indexing
            tunnel: [w70] -> w54 mode=indexing
            n180 = Unbundle By Name(w71) -> ("Name"=w70:string)
          }
          n181 = Greater Than 0?(x=w63) -> (x > 0?=w64:bool)
          n182 = Select(t=0, s=w64, f=-1) -> (s? t:f=w61:i32)
          n183 = property on="Input Event" class="Input Event XCtrl (strict)"("UserFlags"=w54) -> ()  [unwired: 2 in, 2 out]
          n184 = property on="FSM.Graph" class="FSMGraph (strict)"("Events"=w56) -> ()  [unwired: 2 in, 2 out]
          n185 = property on="EventList" class="KListboxEx (strict)"("Items"=w56, "Value"=w61) -> ()  [unwired: 2 in, 2 out]
          n186 = Bundle By Name(cluster=w68, "selectedEvent"=w61) -> (w67:T8)
          n187 = Build Array (concatenate)(w69, "Events.Select") -> (w60:string[])
        }
        frame "Events.Select" {
          n188 = Unbundle By Name(w82) -> ("selectedEvent"=w78:i32)
          n189 = property class="Tosca"(reference=w81) -> ("Accessors:Input Events"=w80:T14[])  [unwired: 1 in, 2 out]
          n190 = Array Size(array=w80) -> (size(s)=w79:i32)
          n191 = Less?(x=w78, y=w79) -> (x < y?=w77:bool)
          n192 = Greater Or Equal To 0?(x=w78) -> (x >= 0?=w76:bool)
          n193 = And(x=w77, y=w76) -> (x .and. y?=w75:bool)
          n194 = case shown="True" w75 {
            tunnel: w80 -> [w86 _]
            tunnel: w78 -> [w84 _]
            frame True {
              n195 = Index Array(array=w86, index=w84) -> (element=w85:T14)
              n196 = property on="Input Event" class="Input Event XCtrl (strict)"("Visible"=TRUE, "Value"=w85) -> ()  [unwired: 2 in, 2 out]
            }
            frame False {
              n197 = property on="Input Event" class="Input Event XCtrl (strict)"("Visible"=FALSE) -> ()  [unwired: 2 in, 2 out]
            }
          }
        }
        frame "General.Show" {
          n198 = property class="Tosca"(reference=w99) -> (reference out=w91:refnum<class "Parameters.lvclass">, "Accessors:DAQ"=w94:T18, "Accessors:Schedule Mode"=w102:T9)  [unwired: 1 in, 1 out]
          n199 = property class="Tosca"(reference=w99) -> ("Accessors:Pretrial"=w98:T19)  [unwired: 1 in, 2 out]
          n200 = Equal?(x=w102, y=Tosca-Schedule_Mode."CS+/CS-" ("Schedule Mode")) -> (x = y?=w100:bool)
          n201 = Unbundle By Name(w98) -> ("Path"=w97:path)
          n202 = local write "DAQ"(w94) -> ()
          n203 = local write "Mode"(w102) -> ()
          n204 = Unbundle By Name(w94) -> ("Poll Rate (Hz)"=w92:dbl)
          n205 = property on="FSM.Graph" class="FSMGraph (strict)"("CS+CS-"=w100) -> ()  [unwired: 2 in, 2 out]
          n206 = Empty String/Path?(string/path=w97) -> (empty?=w96:bool)
          n207 = Not(x=w96) -> (.not. x?=w95:bool)
          n208 = property on="State.Script" class="Bool (strict)"("Visible"=w95) -> ()  [unwired: 2 in, 2 out]
          n209 = Divide(x=1000.0, y=w92) -> (x/y=w90:dbl)
          n210 = property on="SigMan" class="SignalManager (strict)"("Frame (ms)"=w90) -> ()  [unwired: 2 in, 2 out]
          n211 = call "Set Frame Size.vi"("Frame (ms)"=w90, "Tosca in"=w91) -> ("Tosca out"=w89:refnum<class "Parameters.lvclass">)  [unwired: 8 in, 1 out]
        }
        frame "Graph.SelectEdge" {
          n212 = Unbundle By Name(w113) -> ("selectedState"=w110:i32, "selectedTrans"=w107:i32)
          n213 = Unbundle By Name(w113) -> ("termSelected"=w109:bool)
          n214 = property class="Tosca"(reference=w112) -> ("Accessors:Flowchart"=w111:refnum<class "State.lvclass">[])  [unwired: 1 in, 2 out]
          n215 = Index Array(array=w111, index=w110) -> (element=w108:refnum<class "State.lvclass">)
          n216 = case shown="False" w109 {
            tunnel: w108 -> [w122 _]
            tunnel: w107 -> [w121 _]
            frame False {
              n217 = property class="State"(reference=w122) -> ("Accessors:Name"=w118:string, "Accessors:Timeouts"=w120:refnum<class "Timeout.lvclass">[])  [unwired: 1 in, 2 out]
              n218 = Index Array(array=w120, index=w121) -> (element=w119:refnum<class "Timeout.lvclass">)
              n219 = property class="Timeout"(reference=w119) -> ("Accessors:Link to"=w117:string, "Accessors:Type"=w116:T20)  [unwired: 1 in, 2 out]
              n220 = case shown="\"CS-\"" w116 {
                tunnel: ["Any" "CS+" "CS-"] -> w115
                frame "Normal", Default {
                }
                frame "CS+" {
                }
                frame "CS-" {
                }
              }
              n221 = invoke on="FSM.Graph" class="FSMGraph (strict)" method="Select Edge.vi"("From"=w118, "To"=w117, "Type"=w115) -> ()  [unwired: 3 in, 6 out]
            }
            frame True {
            }
          }
        }
        frame "Grating.OnOff" {
          n222 = local read "Grating"() -> (w131:T7)
          n223 = Unbundle By Name(w131) -> ("Grating type"=w130:enum16{"OFF", "Square", "Sine"})
          n224 = Not Equal?(x=w130, y=enum16{"OFF", "Square", "Sine"}."OFF") -> (x != y?=w128:bool)
          n225 = call "Enable or Gray Out.vi"("Boolean"=w128) -> ("Disabled"=w127:T11)
          n226 = property on="Orientation (degrees)" class="DigNum (strict)"("DisabledEnum"=w127) -> ()  [unwired: 2 in, 2 out]
          n227 = property on="Mean intensity (0-1)" class="DigNum (strict)"("DisabledEnum"=w127) -> ()  [unwired: 2 in, 2 out]
          n228 = property on="Spatial frequency (cpd)" class="DigNum (strict)"("DisabledEnum"=w127) -> ()  [unwired: 2 in, 2 out]
          n229 = property on="Phase (cycles)" class="DigNum (strict)"("DisabledEnum"=w127) -> ()  [unwired: 2 in, 2 out]
          n230 = property on="Velocity (Hz)" class="DigNum (strict)"("DisabledEnum"=w127) -> ()  [unwired: 2 in, 2 out]
          n231 = property on="Contrast (0-1)" class="DigNum (strict)"("DisabledEnum"=w127) -> ()  [unwired: 2 in, 2 out]
          n232 = property on="Duration (ms)" class="DigNum (strict)"("DisabledEnum"=w127) -> ()  [unwired: 2 in, 2 out]
        }
        frame "SigMan.Update" {
          # "Don't show fade in"
          n233 = local read "SigMan"() -> (w140:refnum<class "SignalManager.lvclass">)
          n234 = control-ref of="Graph"() -> (w143:refnum<vi>)
          n235 = call "Initialize.vi"("SigMan in"=w140) -> ("error out"=w138:errorcluster, "SigMan out"=w139:refnum<class "SignalManager.lvclass">)  [unwired: 9 in]
          n236 = control-ref of="This VI"() -> (w142:refnum<vi>)
          n237 = call "Tosca-Adjust Laser PWM.vi"("SigMan in"=w139, "error in (no error)"=w138) -> ("SigMan out"=w136:refnum<class "SignalManager.lvclass">, "error out"=w137:errorcluster)  [unwired: 12 in]
          n238 = case shown="No Error" w137 {
            selector: w137 -> [w154 _]
            tunnel: w136 -> [w161 w162]
            tunnel: w143 -> [w158 _]
            tunnel: w142 -> [w157 _]
            tunnel: [w155 _] -> _
            tunnel: [w153 w162] -> w135
            frame No Error {
              n239 = call "Timing-Tick Tock.vi"("error in (no error)"=w154) -> ("error out"=w151:errorcluster)  [unwired: 5 in, 1 out]
              n240 = call "Synthesize.vi"("error in (no error)"=w151, "Repetition"=1, "SigMan in"=w161) -> ("error out"=w156:errorcluster, "Array"=w159:dbl[][], "SigMan out"=w160:refnum<class "SignalManager.lvclass">)  [unwired: 6 in]
              n241 = call "Timing-Tick Tock.vi"("error in (no error)"=w156) -> ("error out"=w150:errorcluster)  [unwired: 5 in, 1 out]
              n242 = call "Plot.vi"("SigMan in"=w160, "Graph"=w158, "VI"=w157, "Array"=w159, "error in (no error)"=w150) -> ("SigMan out"=w153:refnum<class "SignalManager.lvclass">, "error out"=w155:errorcluster)  [unwired: 9 in]
            }
            frame Error {
            }
          }
          n243 = property class="SigMan"(reference=w135) -> ("Accessors:Error"=w146:string)  [unwired: 1 in, 2 out]
          "Error" <- w146
          n244 = Empty String/Path?(string/path=w146) -> (empty?=w144:bool)
          n245 = Boolean To (0,1)(Boolean=w144) -> (0, 1=w145:i16)
          n246 = local write "Sig Tab"(w145) -> ()
        }
        frame "State.EnableTabs" {
          n247 = Unbundle By Name(w174) -> ("selectedState"=w171:i32)
          n248 = property on="Tabs" class="TabCtl (strict)"() -> ("Pages"=w172:refnum<vi>[], "Value"=w164:T1)  [unwired: 2 in, 2 out]
          n249 = Greater Or Equal To 0?(x=w171) -> (x >= 0?=w166:bool)
          n250 = for {
            N: 3 -> [_]
            tunnel: w172 -> [w182]
            tunnel: [w180] -> w170
            tunnel: T10."State" ("Tabs") -> [w179]
            tunnel: w166 -> [w178]
            i -> [w176]
            n251 = Add(x=w179, y=w176) -> (x+y=w177:u32)
            n252 = Index Array(array=w182, index=w177) -> (element=w181:refnum<vi>)
            n253 = property class="Page"(reference=w181, "PageVis"=w178) -> (error out=w180:errorcluster)  [unwired: 1 in, 1 out]
          }
          n254 = Less?(x=w164, y=2) -> (x < y?=w165:bool)
          n255 = case shown="True" w166 {
            tunnel: w170 -> [w184 w186]
            tunnel: w165 -> [_ w185]
            frame False {
              n256 = property on="Tabs" class="TabCtl (strict)"(error in=w184, "Value"=T1."Events" ("Tabs")) -> ()  [unwired: 1 in, 2 out]
            }
            frame True {
              n257 = case shown="True" w185 {
                tunnel: w186 -> [_ w188]
                frame False {
                }
                frame True {
                  n258 = property on="Tabs" class="TabCtl (strict)"(error in=w188, "Value"=T1."State" ("Tabs")) -> ()  [unwired: 1 in, 2 out]
                }
              }
            }
          }
        }
        frame "State.Select" {
          n259 = Unbundle By Name(w193) -> ("selectedState"=w197:i32)
          n260 = property class="Tosca"(reference=w195) -> ("Accessors:Flowchart"=w196:refnum<class "State.lvclass">[])  [unwired: 1 in, 2 out]
          n261 = property class="Tosca"(reference=w195) -> ("Accessors:First state"=w194:string, "Accessors:Target state"=w189:string)  [unwired: 1 in, 2 out]
          n262 = case shown="0, Default" w197 {
            selector: w197 -> [w217 _]
            tunnel: w196 -> [w218 _]
            tunnel: w194 -> [w216 _]
            tunnel: [string[] ["Grating.OnOff", "SigMan.Update", "Transitions.Select"] _] -> w191
            tunnel: [w208 _] -> _
            tunnel: w189 -> [w202 _]
            frame 0, Default {
              n263 = Index Array(array=w218, index=w217) -> (element=w214:refnum<class "State.lvclass">)
              n264 = property class="State"(reference=w214) -> ("Accessors:Name"=w203:string, "Accessors:Execute script"=w199:bool, "Accessors:TTL-only"=w204:bool, "Accessors:SigMan"=w210:refnum<class "SignalManager.lvclass">, "Accessors:Grating"=w211:T21)  [unwired: 1 in, 2 out]
              n265 = local write "Grating"(w211) -> ()
              n266 = call "Initialize.vi"("SigMan in"=w210) -> ("error out"=w208:errorcluster, "SigMan out"=w209:refnum<class "SignalManager.lvclass">)  [unwired: 9 in]
              n267 = Not(x=w204) -> (.not. x?=w212:bool)
              n268 = Equal?(x=w203, y=w216) -> (x = y?=w207:bool)
              n269 = Equal?(x=w203, y=w202) -> (x = y?=w200:bool)
              n270 = local write "State.Name"(w203) -> ()
              n271 = local write "State.Script"(w199) -> ()
              n272 = local write "SigMan"(w209) -> ()
              n273 = Not(x=w207) -> (.not. x?=w206:bool)
              n274 = Or(x=w206, y=w204) -> (x .or. y?=w205:bool)
              n275 = call "Enable or Gray Out.vi"("Boolean"=w212) -> ("Disabled"=w201:T11)
              n276 = call "Enable or Gray Out.vi"("Boolean"=w205) -> ("Disabled"=w215:T11)
              n277 = property on="State.Target" class="Bool (strict)"("Value"=w200, "DisabledEnum"=w201) -> ()  [unwired: 2 in, 2 out]
              n278 = property on="State.Start here" class="Bool (strict)"("Value"=w207, "DisabledEnum"=w215) -> ()  [unwired: 2 in, 2 out]
              n279 = property on="Time/Term" class="TabCtl (strict)"("DisabledEnum"=w201) -> ()  [unwired: 2 in, 2 out]
              n280 = property on="TTL" class="TTL XCtrl (strict)"("DisabledEnum"=w201) -> ()  [unwired: 2 in, 2 out]
            }
            frame -1 {
            }
          }
          n281 = Build Array (concatenate)(w198, w191) -> (w192:string[])
        }
        frame "Transitions.Select" {
          n282 = Unbundle By Name(w229) -> ("selectedState"=w223:i32, "selectedTrans"=w220:i32)
          n283 = Unbundle By Name(w229) -> ("termSelected"=w222:bool)
          n284 = property class="Tosca"(reference=w225) -> ("Accessors:Flowchart"=w224:refnum<class "State.lvclass">[])  [unwired: 1 in, 2 out]
          n285 = Select(t=enum32{"Timeout", "Term"}."Term" ("Time/Term"), s=w222, f=enum32{"Timeout", "Term"}."Timeout" ("Time/Term")) -> (s? t:f=w227:enum32{"Timeout", "Term"})
          n286 = local write "Time/Term"(w227) -> ()
          n287 = Index Array(array=w224, index=w223) -> (element=w221:refnum<class "State.lvclass">)
          n288 = case shown="True" w222 {
            tunnel: w221 -> [w240 w260]
            tunnel: w220 -> [w238 w258]
            frame False {
              n289 = property class="State"(reference=w240) -> ("Accessors:Timeouts"=w239:refnum<class "Timeout.lvclass">[])  [unwired: 1 in, 2 out]
              n290 = Index Array(array=w239, index=w238) -> (element=w235:refnum<class "Timeout.lvclass">)
              n291 = property class="Timeout"(reference=w235) -> (reference out=w236:refnum<class "Timeout.lvclass">, "Accessors:TTL"=w237:refnum<class "TTLController.lvclass">[], "Accessors:Type"=w234:T20)  [unwired: 1 in, 1 out]
              n292 = case shown="\"CS+\"" w234 {
                tunnel: [u32 0 u32 38144 u32 12582912] -> w232
                tunnel: [w241 w244 w248] -> w233
                tunnel: "Timeout" ("Accessors:Source") -> [w241 w245 w247]
                frame "Normal", Default {
                }
                frame "CS+" {
                  n293 = Concatenate Strings(w245, ": CS+" ("string")) -> (w244:string)
                }
                frame "CS-" {
                  n294 = Concatenate Strings(w247, ": CS-" ("string")) -> (w248:string)
                }
              }
              n295 = property on="Timeout" class="Timeout XCtrl (strict)"("Caption.Text"=w233, "Caption.TextColor"=w232) -> ()  [unwired: 2 in, 2 out]
              n296 = local write "Timeout"(w236) -> ()
              n297 = local write "TTL"(w237) -> ()
            }
            frame True {
              n298 = property class="State"(reference=w260) -> ("Accessors:Term"=w259:refnum<class "Termination.lvclass">[])  [unwired: 1 in, 2 out]
              n299 = Index Array(array=w259, index=w258) -> (element=w256:refnum<class "Termination.lvclass">)
              n300 = property class="Term"(reference=w256) -> (reference out=w255:refnum<class "Termination.lvclass">, "Accessors:TTL"=w257:refnum<class "TTLController.lvclass">[], "Accessors:Source"=w253:string, "Accessors:Type"=w254:T20)  [unwired: 1 in, 1 out]
              n301 = case shown="\"CS+\"" w254 {
                tunnel: [u32 0 u32 38144 u32 12582912] -> w251
                tunnel: [w261 w264 w268] -> w252
                tunnel: w253 -> [w261 w265 w267]
                frame "Normal", Default {
                }
                frame "CS+" {
                  n302 = Concatenate Strings(w265, ": CS+" ("string")) -> (w264:string)
                }
                frame "CS-" {
                  n303 = Concatenate Strings(w267, ": CS-" ("string")) -> (w268:string)
                }
              }
              n304 = property on="Term" class="Termination XCtrl (strict)"("Caption.Text"=w252, "Caption.TextColor"=w251) -> ()  [unwired: 2 in, 2 out]
              n305 = local write "Term"(w255) -> ()
              n306 = local write "TTL"(w257) -> ()
            }
          }
        }
        frame "cancel" {
          n307 = Unregister For Events(event registration refnum=w274) -> ()  [unwired: 1 in, 1 out]
          n308 = local read "FSM In"() -> (w271:refnum<class "FSM.Graph.lvclass">)
          n309 = local read "Tosca"() -> (w272:refnum<class "Parameters.lvclass">)
        }
        frame "ok" {
          n310 = Unregister For Events(event registration refnum=w280) -> ()  [unwired: 1 in, 1 out]
          n311 = local read "FSM.Graph"() -> (w279:refnum<class "FSM.Graph.lvclass">)
          n312 = call "Clear Selections.vi"("FSM in"=w279) -> ("FSM out"=w278:refnum<class "FSM.Graph.lvclass">)  [unwired: 9 in, 1 out]
        }
      }
      n313 = Empty Array?(array=w45) -> (empty?=w44:bool)
    }
  }
  "Tosca out" <- w8
  "FSM out" <- w7
  "canceled" <- w6
